vi "General EigenVectors and Values.vi"(3 "output option":T1=1 items=["Eigenvalues", "Eigenvalues & Vectors"], 5 "Input Matrix":T3) -> (0 "error":i32, 1 "Eigenvectors":T2, 2 "Eigenvalues":cdb[](array[numeric]) format="%.2f")   [LabVIEW 2017, in "NI_AALBase.lvlib"]
uses:
  NI_AALBase.lvlib
  RealMatrix.ctl
  ComplexMatrix.ctl
  Eigenvalue and Vectors Output Option.ctl
  lvanlys.dll
  NI_Matrix.lvlib
  NI_AALPro.lvlib
panel:
  # "General EigenVectors and Values"
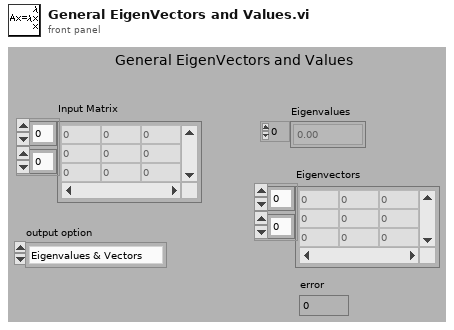
[diagram p1: front panel]
types:
  T1 = typedef "NI_AALPro.lvlib/Eigenvalue and Vectors Output Option.ctl" = i32
  T2 = typedef "NI_Matrix.lvlib/ComplexMatrix.ctl" = cdb[][]
  T3 = typedef "NI_Matrix.lvlib/RealMatrix.ctl" = dbl[][]
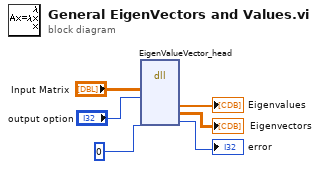
[diagram p0: block diagram]
diagram:
  n1 = dll-call lib="C:/Program Files/National Instruments/LabVIEW 2017/resource/lvanlys.*" fn="EigenValueVector_head"("Input Matrix"="Input Matrix", "output option"="output option", 0) -> ("Eigenvalues"=→"Eigenvalues":cdb[], "Eigenvectors"=→"Eigenvectors":T2, →"error":i32)  [unwired: 8 in, 2 out]
